vi "Open Playback Files Data Recorder.vi"(8 "error in (no error)":errorcluster, 11 "Frame Grabber Data In":T2={"Camera Session"="", "Frame"=refnum, "AVI Refnum"=refnum, "Codecs"=[], "Frame number"=0, "Tracking File Refnum"=refnum, "Tick Count"=0, "Probe Object"=refnum, "Playback Probe Data"=[], "Rigid Body"={"Position"={"x (mm)"=0.0, "y (mm)"=0.0, "z (mm)"=0.0}, "Orientation"={"Pitch (rad)"=0.0, "Yaw (rad)"=0.0, "Roll (rad)"=0.0}, "Quaternion"={"qx"=0.0, "qy"=0.0, "qz"=0.0, "qw"=0.0}, "Tracked?"=FALSE}, "Total no frames playback"=0, "Video FPS"=0.0, "Camera connected?"=FALSE, "Scene"=refnum, "Cropped Frame"=refnum, "Tracker FPS"=0.0, "Crop ROI"=[], "Presentation Values"=[], "Elapsed time (ms)"=0, "Camera frames playback"=0, "Refnums"={"Live Refnum"=refnum, "Record Refnum"=refnum, "Playback Refnum"=refnum, "Frame Slider Refnum"=refnum, "Pause Refnum"=refnum, "Home Refnum"=refnum, "Set Crop Refnum"=refnum, "Clear Crop Refnum"=refnum, "stop refnum"=refnum, "Playback Rate Refnum"=refnum, "Presentation Refnum"=refnum, "Crop Time Frame Slider Refnum"=refnum, "Cancel Save Refnum"=refnum, "Reverse Playback Refnum"=refnum, "Recording Settings Refnum"=refnum, "Continuous Playback Refnum"=refnum, "Camera Frame Refnum"=refnum, "Annotation Refnum"=refnum, "Export All Refnum"=refnum, "Export List Refnum"=refnum, "Fill List Refnum"=refnum, "Save Crop Refnum"=refnum, "Skip Forward Refnum"=refnum, "Skip Backward Refnum"=refnum, "Single Annotation Refnum"=refnum, "Load Refnum"=refnum, "Set Start Refnum"=refnum, "Set End Refnum"=refnum, "Add to List Refnum"=refnum, "List of Annotations Refnum"=refnum}, "Dimensions"={"Probe Dimensions"={"Probe Width"=0.0, "Probe Depth"=1.0, "Probe Height"=0.0}, "Room Dimensions"={"Room Width"=0.0, "Room Depth"=0.0, "Room Height"=0.0}}, "Playback Data As Strings"=[], "Cropped Tracking File Refnum"=refnum, "Cropped AVI Refnum"=refnum, "Header"=[], "Total euclidian distance"=0.0, "Annotation File Path"=path "", "Playback File Path"=path "", "Size per frame"=0.0, "Ground Truth File Refnum"=refnum, "Annotation Array"=[], "Annotation TIFFs Folder"=path ""}) -> (0 "error out":errorcluster, 1 "Playback Video":path, 2 "both exist and open?":bool, 3 "Frame Grabber Data Out":T2={"Camera Session"="", "Frame"=refnum, "AVI Refnum"=refnum, "Codecs"=[], "Frame number"=0, "Tracking File Refnum"=refnum, "Tick Count"=0, "Probe Object"=refnum, "Playback Probe Data"=[], "Rigid Body"={"Position"={"x (mm)"=0.0, "y (mm)"=0.0, "z (mm)"=0.0}, "Orientation"={"Pitch (rad)"=0.0, "Yaw (rad)"=0.0, "Roll (rad)"=0.0}, "Quaternion"={"qx"=0.0, "qy"=0.0, "qz"=0.0, "qw"=0.0}, "Tracked?"=FALSE}, "Total no frames playback"=0, "Video FPS"=0.0, "Camera connected?"=FALSE, "Scene"=refnum, "Cropped Frame"=refnum, "Tracker FPS"=0.0, "Crop ROI"=[], "Presentation Values"=[], "Elapsed time (ms)"=0, "Camera frames playback"=0, "Refnums"={"Live Refnum"=refnum, "Record Refnum"=refnum, "Playback Refnum"=refnum, "Frame Slider Refnum"=refnum, "Pause Refnum"=refnum, "Home Refnum"=refnum, "Set Crop Refnum"=refnum, "Clear Crop Refnum"=refnum, "stop refnum"=refnum, "Playback Rate Refnum"=refnum, "Presentation Refnum"=refnum, "Crop Time Frame Slider Refnum"=refnum, "Cancel Save Refnum"=refnum, "Reverse Playback Refnum"=refnum, "Recording Settings Refnum"=refnum, "Continuous Playback Refnum"=refnum, "Camera Frame Refnum"=refnum, "Annotation Refnum"=refnum, "Export All Refnum"=refnum, "Export List Refnum"=refnum, "Fill List Refnum"=refnum, "Save Crop Refnum"=refnum, "Skip Forward Refnum"=refnum, "Skip Backward Refnum"=refnum, "Single Annotation Refnum"=refnum, "Load Refnum"=refnum, "Set Start Refnum"=refnum, "Set End Refnum"=refnum, "Add to List Refnum"=refnum, "List of Annotations Refnum"=refnum}, "Dimensions"={"Probe Dimensions"={"Probe Width"=0.0, "Probe Depth"=1.0, "Probe Height"=0.0}, "Room Dimensions"={"Room Width"=0.0, "Room Depth"=0.0, "Room Height"=0.0}}, "Playback Data As Strings"=[], "Cropped Tracking File Refnum"=refnum, "Cropped AVI Refnum"=refnum, "Header"=[], "Total euclidian distance"=0.0, "Annotation File Path"=path "", "Playback File Path"=path "", "Size per frame"=0.0, "Ground Truth File Refnum"=refnum, "Annotation Array"=[], "Annotation TIFFs Folder"=path ""})   [LabVIEW 2017]
uses:
  Controls/Frame Grabber Data.ctl
  <vilib>/userdefined/High Color/IMAQdx.ctl
  <vilib>/vision/Image Controls.llb/IMAQ Image.ctl
  <vilib>/vision/Avi.llb/IMAQ AVI2 Refnum.ctl
  Controls/Rigid Body Info.ctl
  Controls/Position.ctl
  Controls/Orientation.ctl
  Controls/Refnums.ctl
  Controls/Recording Settings.ctl
  Controls/Operator Settings.ctl
  Controls/Operator.ctl
  Controls/Patient Settings.ctl
  Controls/Dimensions.ctl
  Controls/Room Dimensions.ctl
panel:
  in  "Operator":T1 items=["Novice", "Expert"]
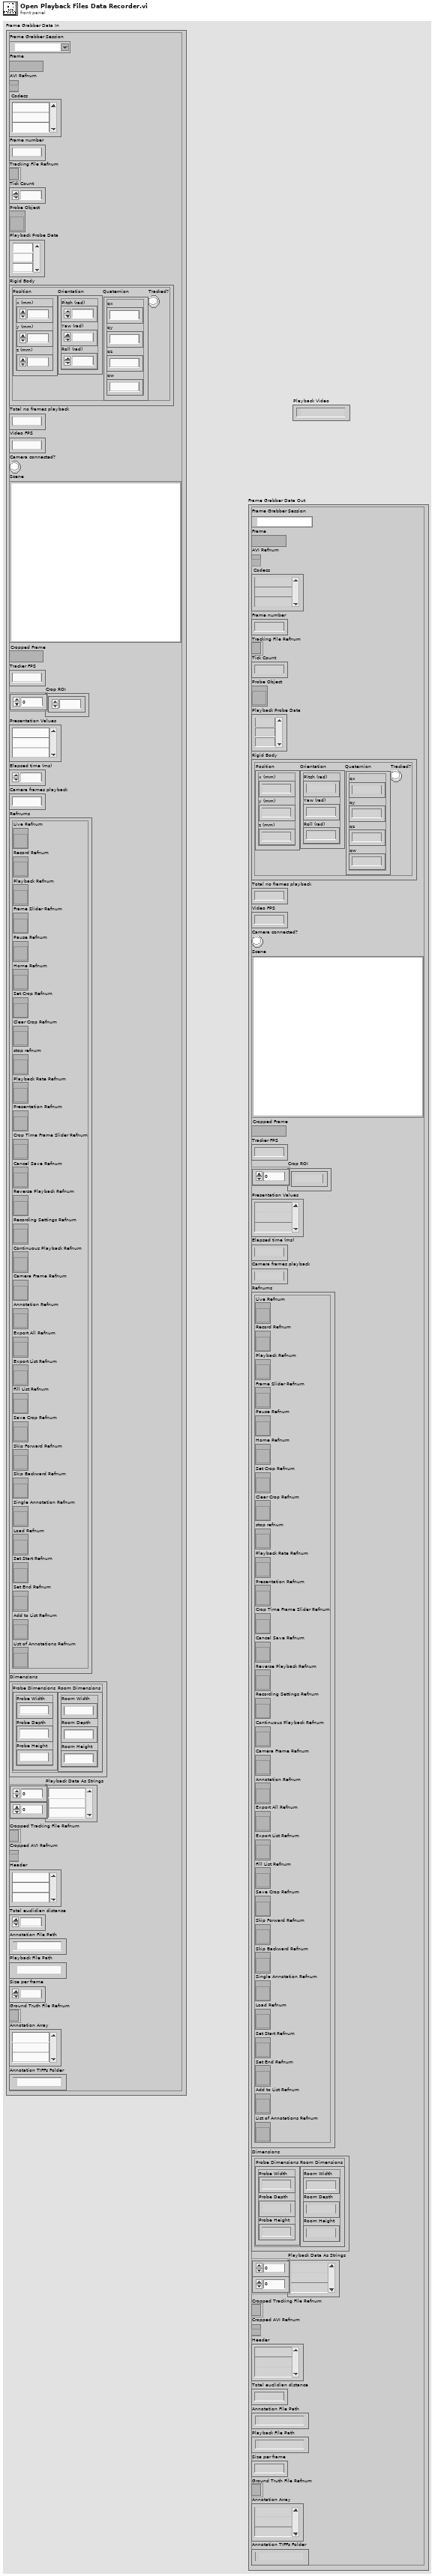
[diagram p1: front panel]
types:
  T1 = typedef "Operator.ctl" = u16
  T2 = typedef "Frame Grabber Data.ctl" = cluster{"Camera Session":T3, "Frame":T4, "AVI Refnum":T5, "Codecs":string[], "Frame number":u32, "Tracking File Refnum":refnum<file>, "Tick Count":u32, "Probe Object":refnum<vi>, "Playback Probe Data":dbl[][], "Rigid Body":T6, "Total no frames playback":i32, "Video FPS":dbl, "Camera connected?":bool, "Scene":refnum<vi>, "Cropped Frame":T4, "Tracker FPS":dbl, "Crop ROI":i32[], "Presentation Values":string[], "Elapsed time (ms)":u32, "Camera frames playback":u32, "Refnums":T9, "Dimensions":T10, "Playback Data As Strings":string[][], "Cropped Tracking File Refnum":refnum<file>, "Cropped AVI Refnum":T5, "Header":string[], "Total euclidian distance":dbl, "Annotation File Path":path, "Playback File Path":path, "Size per frame":dbl, "Ground Truth File Refnum":refnum<file>, "Annotation Array":string[], "Annotation TIFFs Folder":path}
  T3 = typedef "IMAQdx.ctl" = refnum<k21>
  T4 = typedef "IMAQ Image.ctl" = refnum<image>
  T5 = typedef "IMAQ AVI2 Refnum.ctl" = refnum<k20>
  T6 = typedef "Rigid Body Info.ctl" = cluster{"Position":T7, "Orientation":T8, "Quaternion":cluster{"qx":sgl, "qy":sgl, "qz":sgl, "qw":sgl}, "Tracked?":bool}
  T7 = typedef "Position.ctl" = cluster{"x (mm)":sgl, "y (mm)":sgl, "z (mm)":sgl}
  T8 = typedef "Orientation.ctl" = cluster{"Pitch (rad)":sgl, "Yaw (rad)":sgl, "Roll (rad)":sgl}
  T9 = typedef "Refnums.ctl" = cluster{"Live Refnum":refnum<vi>, "Record Refnum":refnum<vi>, "Playback Refnum":refnum<vi>, "Frame Slider Refnum":refnum<vi>, "Pause Refnum":refnum<vi>, "Home Refnum":refnum<vi>, "Set Crop Refnum":refnum<vi>, "Clear Crop Refnum":refnum<vi>, "stop refnum":refnum<vi>, "Playback Rate Refnum":refnum<vi>, "Presentation Refnum":refnum<vi>, "Crop Time Frame Slider Refnum":refnum<vi>, "Cancel Save Refnum":refnum<vi>, "Reverse Playback Refnum":refnum<vi>, "Recording Settings Refnum":refnum<vi>, "Continuous Playback Refnum":refnum<vi>, "Camera Frame Refnum":refnum<vi>, "Annotation Refnum":refnum<vi>, "Export All Refnum":refnum<vi>, "Export List Refnum":refnum<vi>, "Fill List Refnum":refnum<vi>, "Save Crop Refnum":refnum<vi>, "Skip Forward Refnum":refnum<vi>, "Skip Backward Refnum":refnum<vi>, "Single Annotation Refnum":refnum<vi>, "Load Refnum":refnum<vi>, "Set Start Refnum":refnum<vi>, "Set End Refnum":refnum<vi>, "Add to List Refnum":refnum<vi>, "List of Annotations Refnum":refnum<vi>}
  T10 = typedef "Dimensions.ctl" = cluster{"Probe Dimensions":cluster{"Probe Width":sgl, "Probe Depth":sgl, "Probe Height":sgl}, "Room Dimensions":T11}
  T11 = typedef "Room Dimensions.ctl" = cluster{"Room Width":dbl, "Room Depth":dbl, "Room Height":dbl}
  T12 = enum16{"open", "replace", "create", "open or create", "replace or create", "replace or create with confirmation"}
  T13 = cluster{"Width":u32, "Height":u32, "Frames Per Second":u32, "Codec":string, "Has Data":bool}
  T14 = typedef "Recording Settings.ctl" = cluster{"Folder to Save Recordings":path, "Video FPS":u32, "Codec":u16, "Tracker FPS":u32, "Operator ID":T15, "Patient ID/Gestation":T16}
  T15 = typedef "Operator Settings.ctl" = cluster{"Operator ID":u32, "Expertise":T1}
  T16 = typedef "Patient Settings.ctl" = cluster{"ID":u32, "Gestation":string}
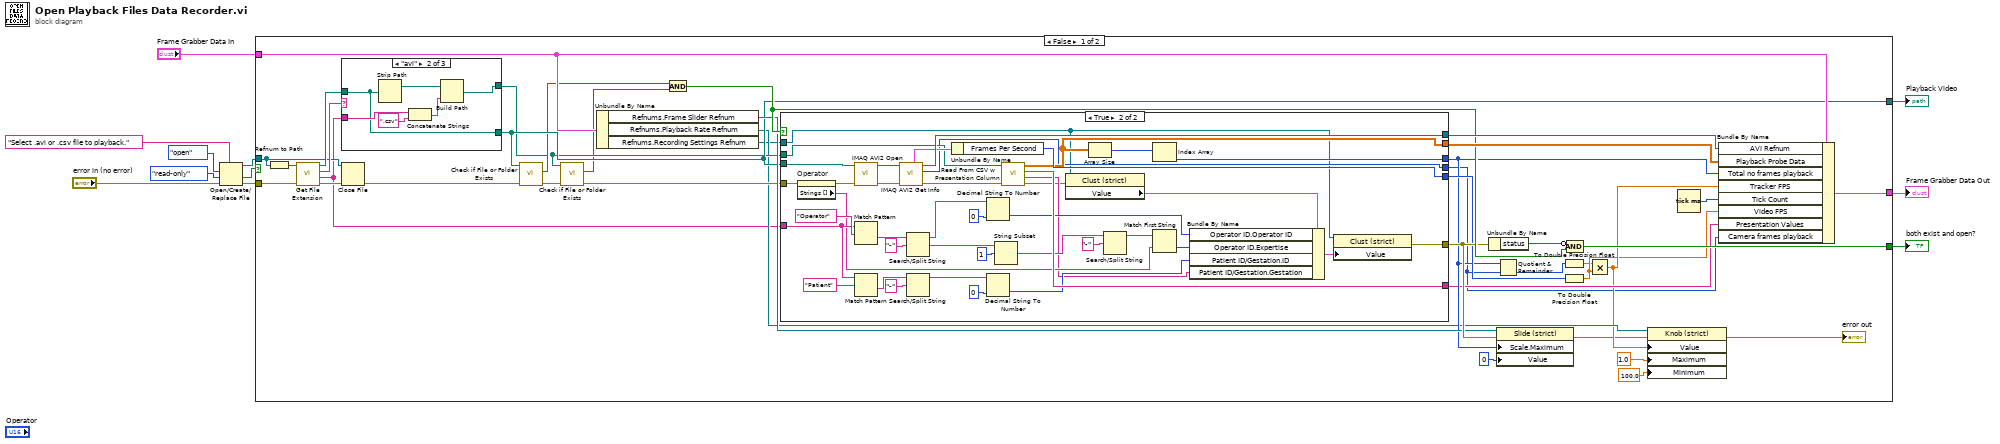
[diagram p0: block diagram]
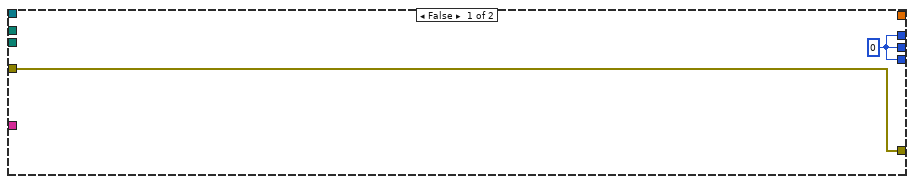
[diagram p2: hidden frame]
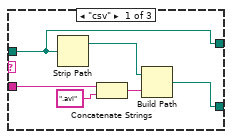
[diagram p3: hidden frame]
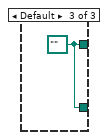
[diagram p4: hidden frame]
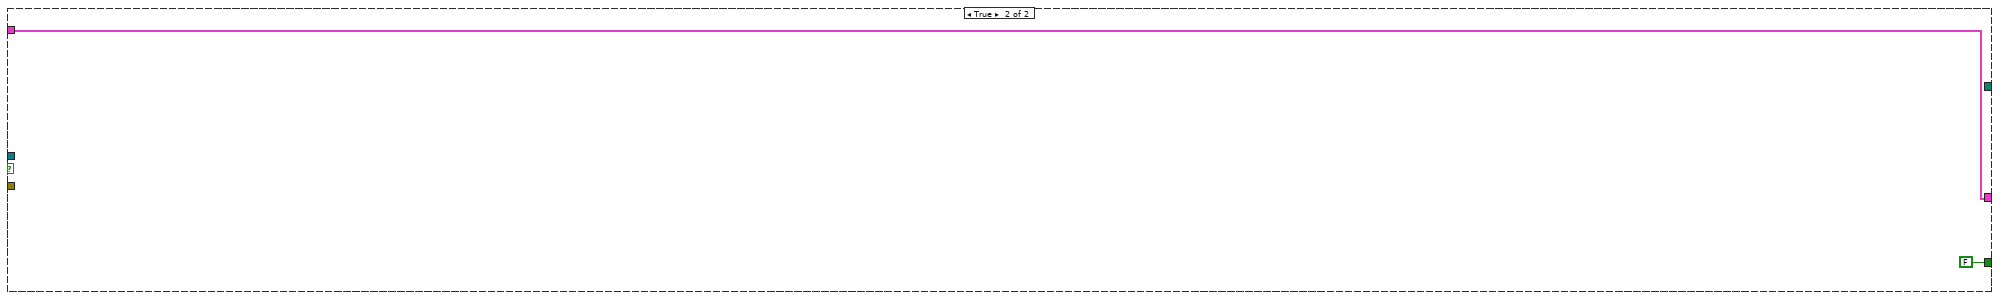
[diagram p5: hidden frame]
diagram:
  n1 = Open/Create/Replace File(error in="error in (no error)", prompt="Select .avi or .csv file to playback.", operation (0:open)=T12."open", access (0:read/write)=enum16{"read/write", "read-only", "write-only"}."read-only") -> (refnum out=w9:refnum<file>, cancelled=w2:bool, error out=w11:errorcluster)  [unwired: 2 in]
  n2 = case shown="False" w2 {
    tunnel: w11 -> [w14 _]
    tunnel: w9 -> [w33 _]
    tunnel: "Frame Grabber Data In" -> [w39 w108]
    tunnel: [w44 FALSE] -> w4
    tunnel: [w42 w108] -> w3
    tunnel: [w29 _] -> w1
    frame False {
      n3 = Refnum to Path(1:w33) -> (0:w50:path)
      n4 = call <vilib>:"Get File Extension.vi"("error in (no error)"=w14, "file"=w50) -> ("error out"=w34:errorcluster, "filename without extension"=w13:string, "lowercase file extension"=w49:string, "dup file"=w48:path)  [unwired: 5 in, 1 out]
      n5 = case shown="\"avi\"" w49 {
        tunnel: w13 -> [w99 w104 _]
        tunnel: w48 -> [w96 w103 _]
        tunnel: [w94 w103 w106] -> w29
        tunnel: [w96 w100 w106] -> w26
        frame "csv" {
          n6 = Strip Path(path=w96) -> (stripped path=w97:path)  [unwired: 1 out]
          n7 = Concatenate Strings(w99, ".avi" ("string")) -> (w95:string)
          n8 = Build Path(base path=w97, name or relative path=w95) -> (appended path=w94:path)
        }
        frame "avi" {
          n9 = Strip Path(path=w103) -> (stripped path=w102:path)  [unwired: 1 out]
          n10 = Concatenate Strings(w104, ".csv" ("string")) -> (w101:string)
          n11 = Build Path(base path=w102, name or relative path=w101) -> (appended path=w100:path)
        }
        frame Default {
          w106 = path "" ("dup file")
        }
      }
      n12 = Close File(refnum=w33, error in=w34) -> (error out=w30:errorcluster)  [unwired: 1 out]
      n13 = call <vilib>:"Check if File or Folder Exists.vi"("error in (no error)"=w30, "path"=w29) -> ("error out"=w24:errorcluster, "file or folder exists?"=w28:bool)  [unwired: 7 in, 1 out]
      n14 = call <vilib>:"Check if File or Folder Exists.vi"("error in (no error)"=w24, "path"=w26) -> ("error out"=w27:errorcluster, "file or folder exists?"=w25:bool)  [unwired: 7 in, 1 out]
      n15 = Unbundle By Name(w39) -> ("Refnums.Frame Slider Refnum"=w38:refnum<vi>, "Refnums.Playback Rate Refnum"=w23:refnum<vi>, "Refnums.Recording Settings Refnum"=w12:refnum<vi>)
      n16 = And(x=w28, y=w25) -> (x .and. y?=w45:bool)
      n17 = case shown="True" w45 {
        tunnel: w27 -> [w52 w79]
        tunnel: w29 -> [_ w93]
        tunnel: [w52 w53] -> w40
        tunnel: [_ w90] -> w47
        tunnel: [_ w87] -> w46
        tunnel: w26 -> [_ w83]
        tunnel: [w51 w81] -> w18
        tunnel: [w51 w88] -> w35
        tunnel: [w51 w84] -> w32
        tunnel: [_ w82] -> w31
        tunnel: w13 -> [_ w77]
        tunnel: w12 -> [_ w69]
        frame False {
          w51 = 0 ("Number of Frames")
        }
        frame True {
          n18 = property on="Operator" class="Ring (strict)"(error in=w79) -> (error out=w55:errorcluster, "Strings []"=w65:string[])  [unwired: 1 in, 1 out]
          n19 = call "IMAQ AVI2 Open"("error in (no error)"=w55, "AVI File Path"=w93) -> ("error out"=w92:errorcluster, "AVI Refnum"=w91:T5)  [unwired: 8 in]
          n20 = Match Pattern(string=w77, regular expression="Operator" ("search string/char (-)")) -> (after substring=w67:string)  [unwired: 1 in, 3 out]
          n21 = Match Pattern(string=w77, regular expression="Patient" ("search string/char (-)")) -> (after substring=w75:string)  [unwired: 1 in, 3 out]
          n22 = call "IMAQ AVI2 Get Info"("error in (no error)"=w92, "AVI Refnum"=w91) -> ("error out"=w86:errorcluster, "Number of Frames"=w81:u32, "AVI Refnum (duplicate)"=w90:T5, "Frame Data"=w89:T13)  [unwired: 5 in, 1 out]
          n23 = Search/Split String(string=w67, search string/char (-)="-") -> (substring before match=w63:string, match + rest of string=w62:string)  [unwired: 1 in, 1 out]
          n24 = Search/Split String(string=w75, search string/char (-)="-") -> (substring before match=w74:string)  [unwired: 1 in, 2 out]
          n25 = Unbundle By Name(w89) -> ("Frames Per Second"=w88:u32)
          n26 = Decimal String To Number(string=w63, default (0L)=u32 0 ("default (0 I32)")) -> (number=w57:u32)  [unwired: 1 in, 1 out]
          n27 = Decimal String To Number(string=w74, default (0L)=u32 0 ("default (0 I32)")) -> (number=w72:u32)  [unwired: 1 in, 1 out]
          n28 = String Subset(string=w62, offset (0)=1) -> (substring=w59:string)  [unwired: 1 in]
          n29 = call "Read From CSV w Presentation Column.vi"("Error In"=w86, "Spreadsheet path (.csv)"=w83) -> ("Error Out"=w54:errorcluster, "Gestation"=w56:string, "Presentation Values"=w82:string[], "Data"=w87:dbl[][])  [unwired: 6 in]
          n30 = property class="Clust (strict)"(reference=w69, error in=w54) -> ("Value"=w71:T14)  [unwired: 2 out]
          n31 = Array Size(array=w87) -> (size(s)=w85:i32[])
          n32 = Search/Split String(string=w59, search string/char (-)="-") -> (substring before match=w58:string)  [unwired: 1 in, 2 out]
          n33 = Index Array(array=w85) -> (element=w84:i32)  [unwired: 1 in]
          n34 = Match First String(2:w65, 3:w58) -> (0:w64:i32)  [unwired: 1 out]
          n35 = Bundle By Name(cluster=w71, "Operator ID.Operator ID"=w57, "Operator ID.Expertise"=w64, "Patient ID/Gestation.ID"=w72, "Patient ID/Gestation.Gestation"=w56) -> (w70:T14)
          n36 = property class="Clust (strict)"(reference=w69, "Value"=w70) -> (error out=w53:errorcluster)  [unwired: 1 in, 1 out]
        }
      }
      n37 = Unbundle By Name(w40) -> ("status"=w43:bool)
      n38 = Quotient & Remainder(x=w32, y=w18) -> (floor(x/y)=w36:u32)  [unwired: 1 out]
      n39 = property class="Slide (strict)"(reference=w38, error in=w40, "Scale.Maximum"=w32, "Value"=u32 0 ("Frame number")) -> (error out=w21:errorcluster)  [unwired: 1 out]
      n40 = To Double Precision Float(number=w36) -> (double precision float=w16:dbl)
      n41 = To Double Precision Float(number=w35) -> (double precision float=w17:dbl)
      n42 = Compound Arithmetic op=AND(invert w43, w45) -> (w44:bool)
      n43 = Multiply(x=w16, y=w17) -> (x*y=w22:dbl)
      n44 = property class="Knob (strict)"(reference=w23, error in=w21, "Value"=w22, "Maximum"=1.0 ("Data Entry Limits:Maximum"), "Minimum"=100.0 ("Data Entry Limits:Minimum")) -> (error out=→"error out":errorcluster)  [unwired: 1 out]
      n45 = Tick Count (ms)() -> (millisecond timer value=w41:u32)
      n46 = Bundle By Name(cluster=w39, "AVI Refnum"=w47, "Playback Probe Data"=w46, "Total no frames playback"=w32, "Tracker FPS"=w22, "Tick Count"=w41, "Video FPS"=w17, "Presentation Values"=w31, "Camera frames playback"=w18) -> (w42:T2)
    }
    frame True {
    }
  }
  "both exist and open?" <- w4
  "Frame Grabber Data Out" <- w3
  "Playback Video" <- w1
